vi "Configuration Window.vi"(8 "error in (no error)":errorcluster, 11 "Inst.TC":refnum<class "Inst.TC.lvclass">) -> (0 "error out":errorcluster, 3 "Inst.TC out":refnum<class "Inst.TC.lvclass">)   [LabVIEW 2019, in "Inst.TC.lvclass"]
uses:
  Inst.TC.lvclass
  C:/Program Files (x86)/National Instruments/LabVIEW 2019/vi.lib/JKI/JKI SMO/SMO/SMO.lvclass
  Inst.TC.lvclass/Inst.TC.ctl
  FP-TC-Shared/FP-TC-Shared.lvclass/FP-TC-Shared.ctl
  <userlib>/LevyLab/Debug/Attribute.Debug/DebugBehavior.ctl
  FP-TC-Shared/FP-TC-Shared.lvclass
  <userlib>/LevyLab/Debug/Debug.lvlib
  <userlib>/LevyLab/Debug/Attribute.Debug/Attribute.Debug.lvclass
panel:
  in  "Debug Mode? [F]":bool
  in  "Paths":string
  in  "LC Type":u16(ring) items=["CF_TC", "CF_TC_Z", "MNK_TC", "MNK_TC_Z"]
  in  "Cancel":bool
  in  "OK":bool
  # "Confirm or Make Changes:"
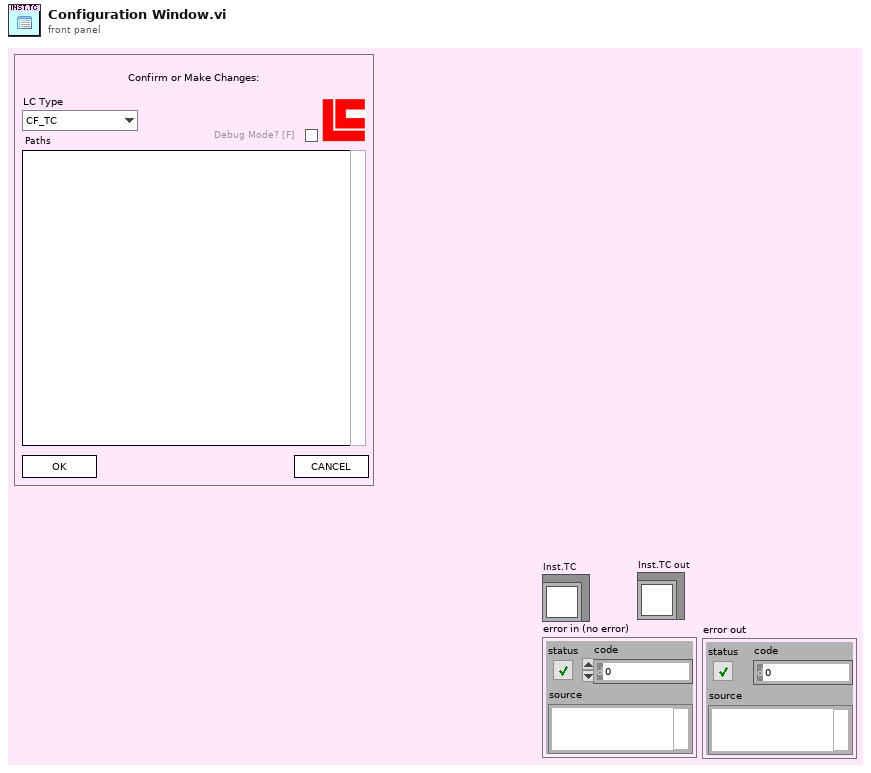
[diagram p1: front panel]
types:
  T1 = enum32{"Invalid", "Standard", "Closed", "Hidden", "Minimized", "Maximized"}
  T2 = enum32{"invalid app kind", "Development System", "Run Time System", "Student Edition", "Embedded LabVIEW", "Evaluation", "Custom"}
  T3 = typedef "Debug.lvlib/Attribute.Debug.lvclass/DebugBehavior.ctl" = enum16{"Normal", "Debug"}
  T4 = cluster{"Core":cluster{"Current VI Reference":refnum<vi>, "Close Panel on Exit?":bool}, "Inst.TC":refnum<class "Inst.TC.lvclass">}
  T5 = typedef "FP-TC-Shared.lvclass/LC Type--Enum.ctl" = enum16{"CF_FP", "CF_TC", "CF_TC_Z", "MNK_FP", "MNK_TC", "MNK_TC_Z", "unknown"}
  T6 = cluster{"Current VI Reference":refnum<vi>, "Close Panel on Exit?":bool}
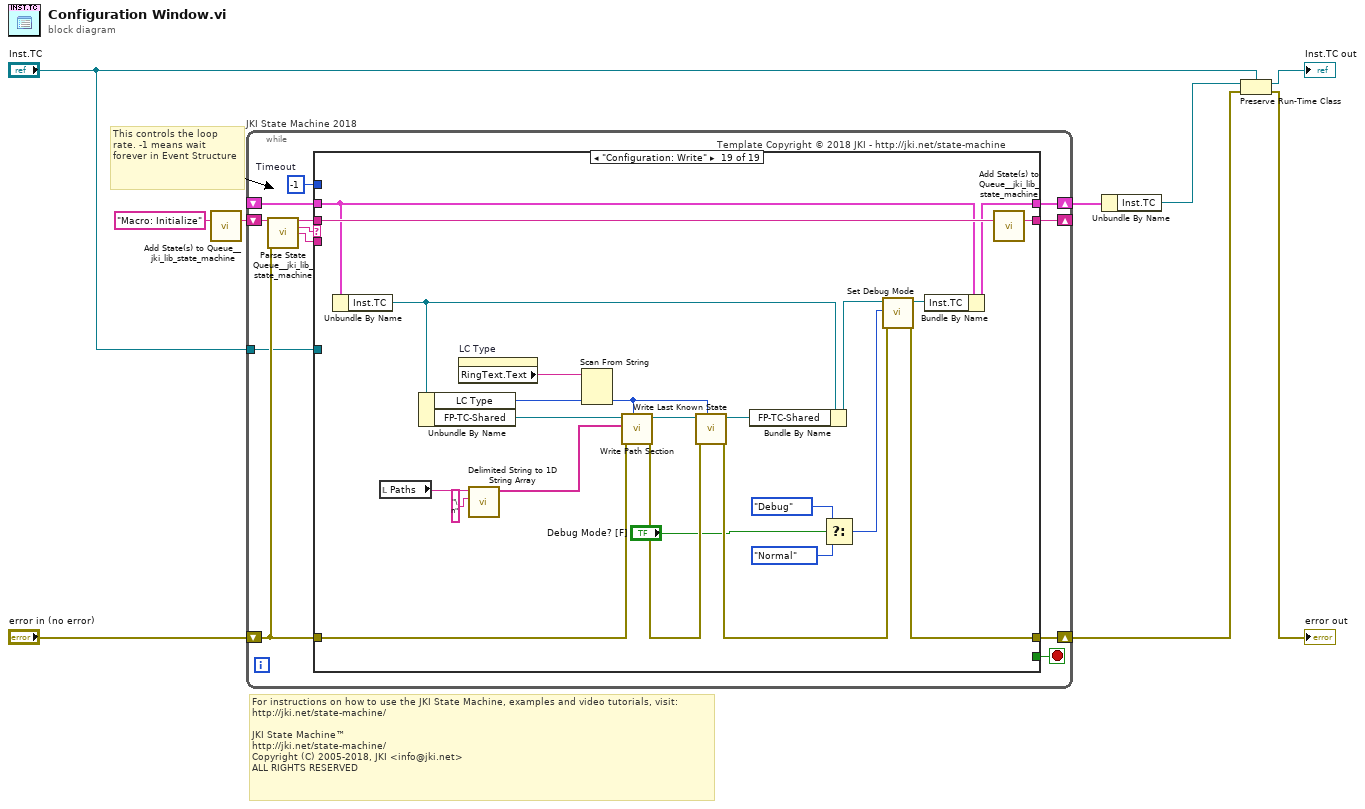
[diagram p0: block diagram]
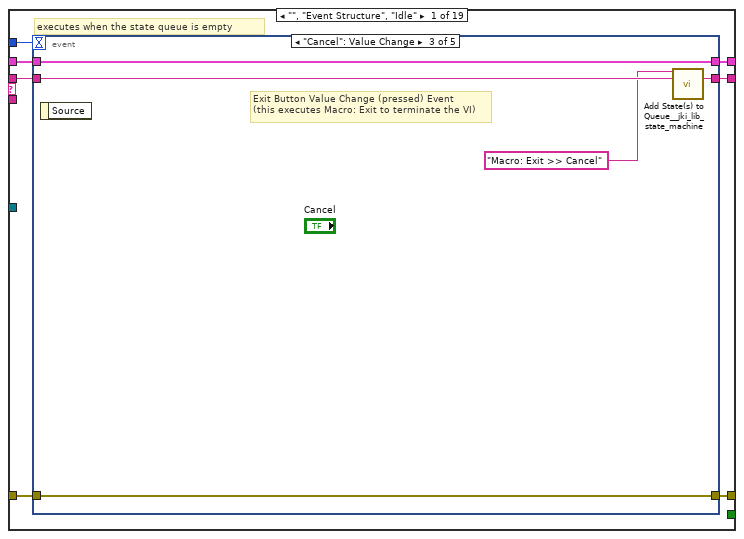
[diagram p2: hidden frame]
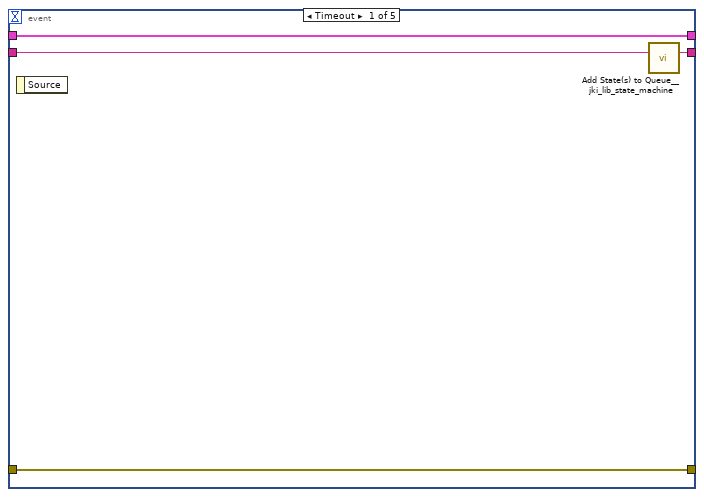
[diagram p3: hidden frame]
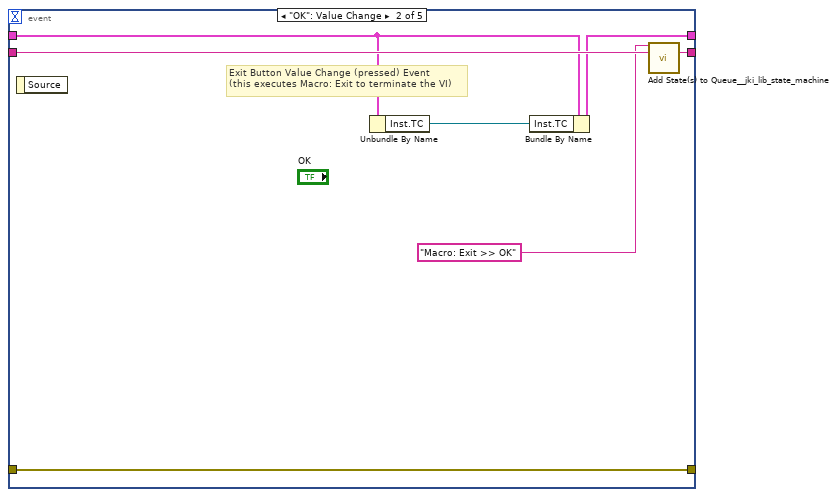
[diagram p4: hidden frame]
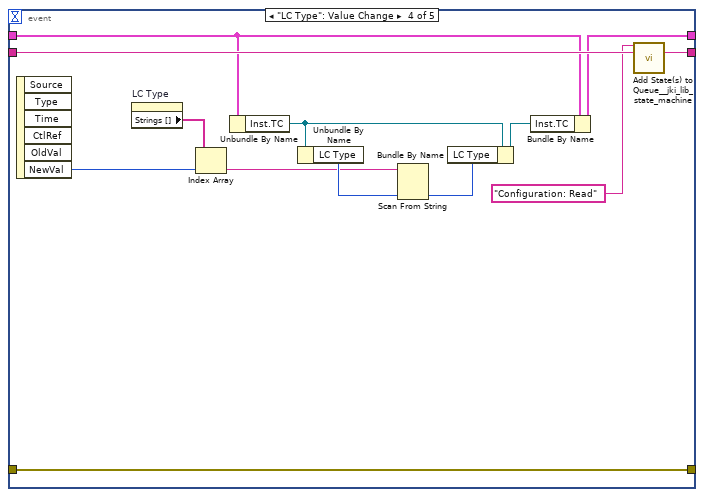
[diagram p5: hidden frame]
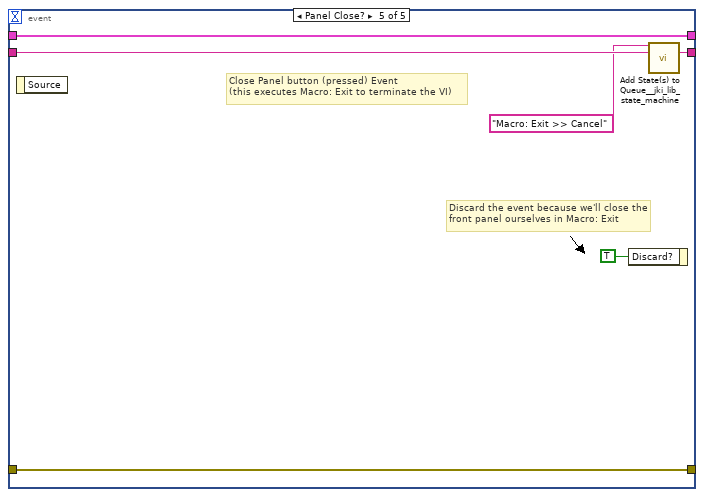
[diagram p6: hidden frame]
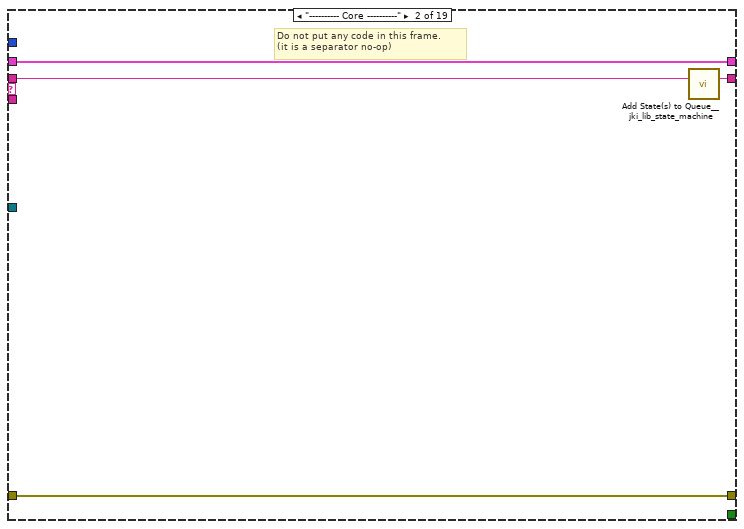
[diagram p7: hidden frame]
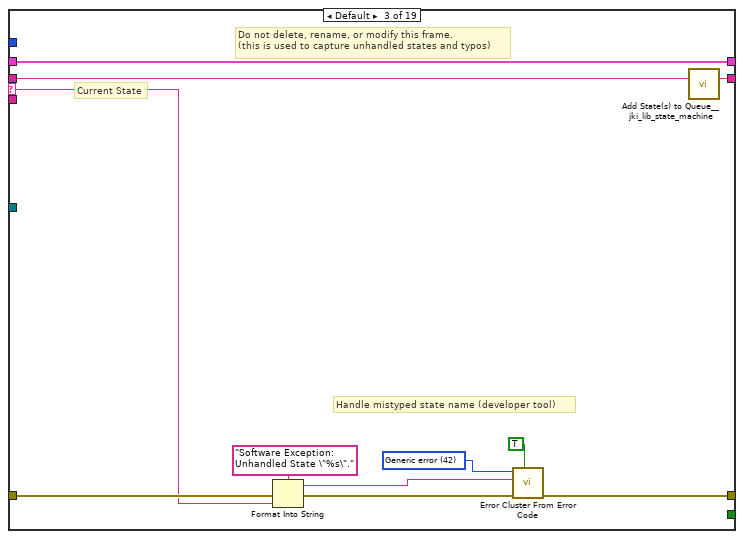
[diagram p8: hidden frame]
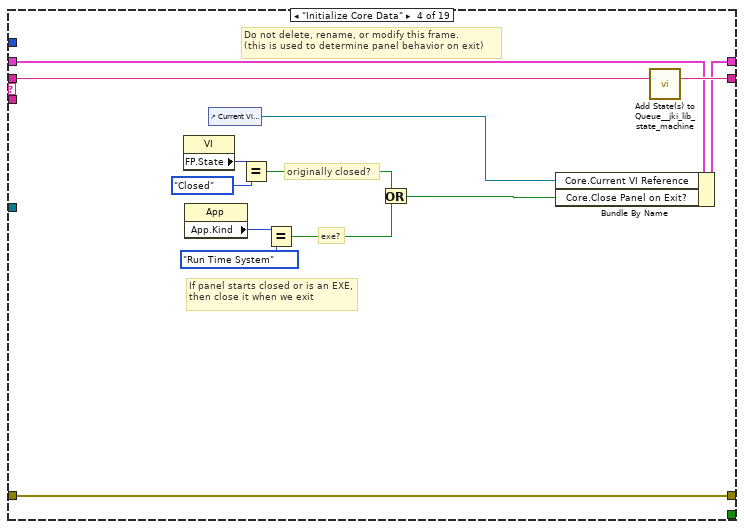
[diagram p9: hidden frame]
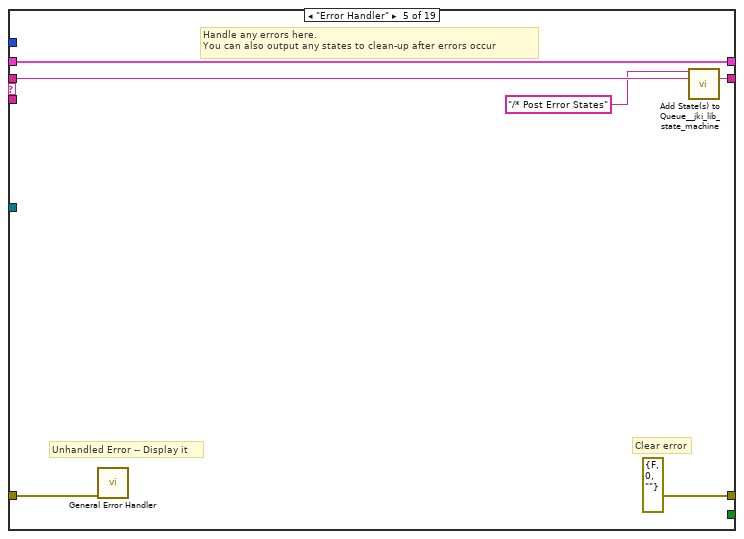
[diagram p10: hidden frame]
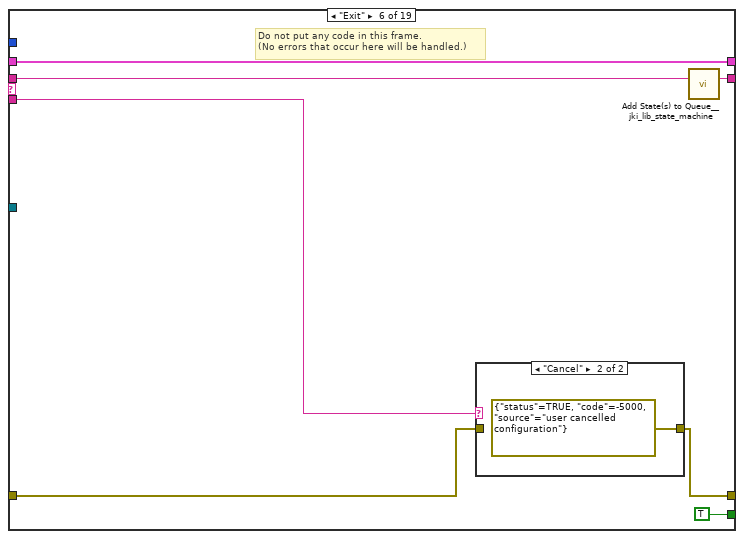
[diagram p11: hidden frame]
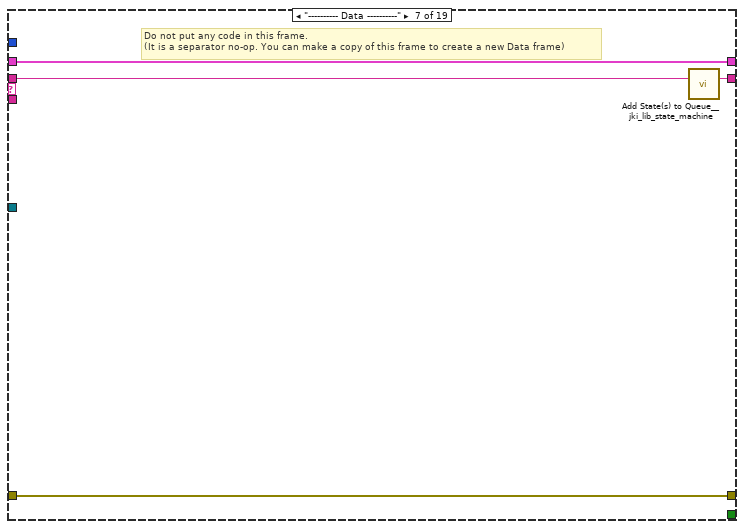
[diagram p13: hidden frame]
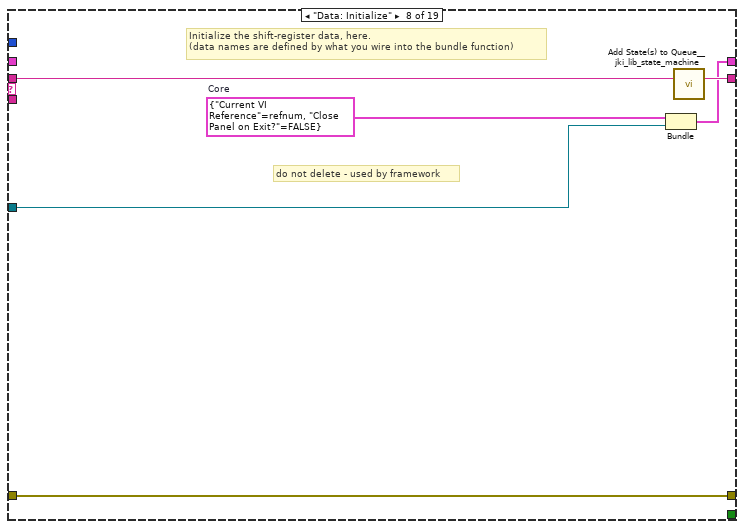
[diagram p14: hidden frame]
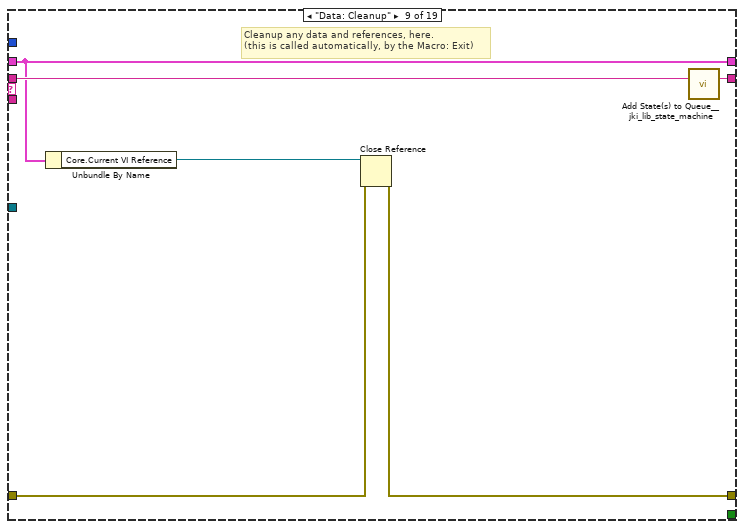
[diagram p15: hidden frame]
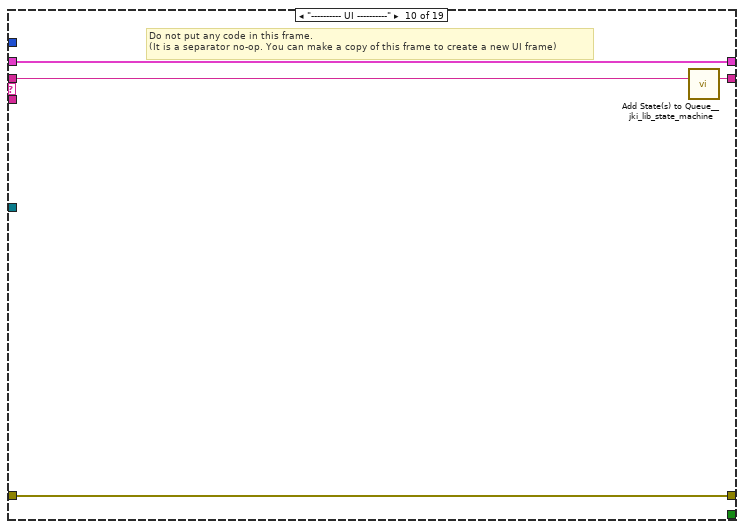
[diagram p16: hidden frame]
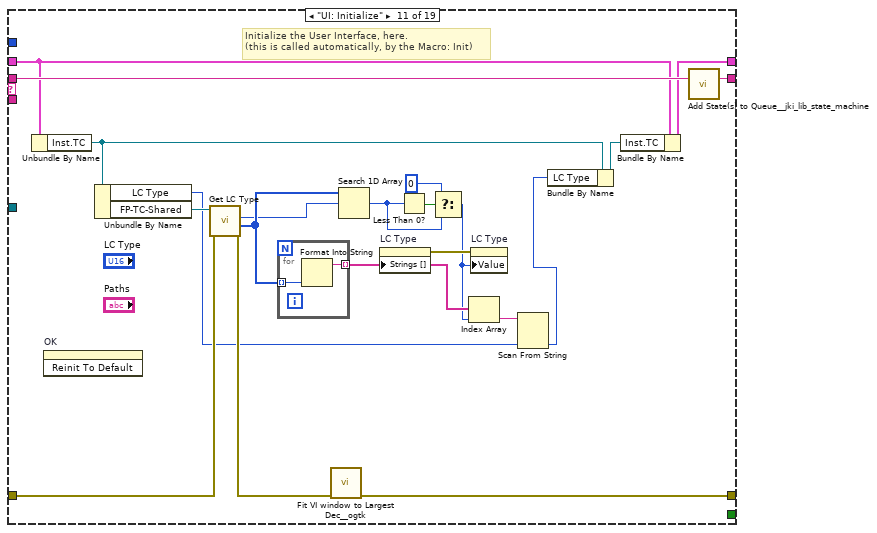
[diagram p17: hidden frame]
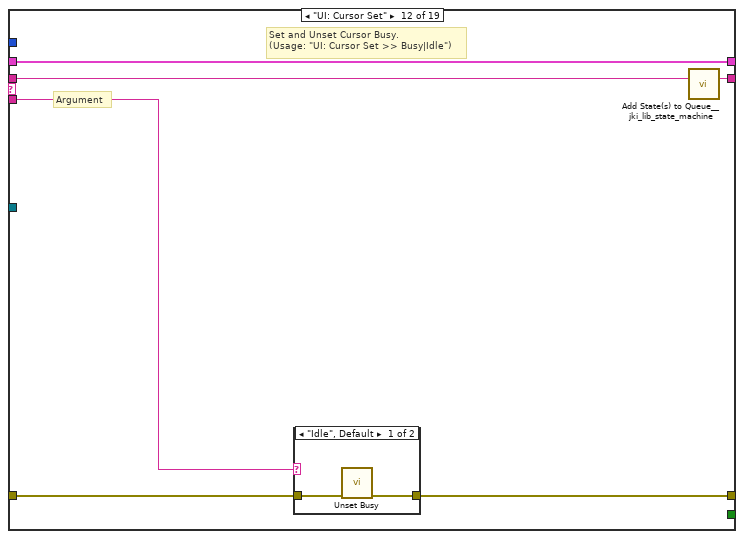
[diagram p18: hidden frame]
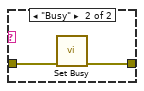
[diagram p19: hidden frame]
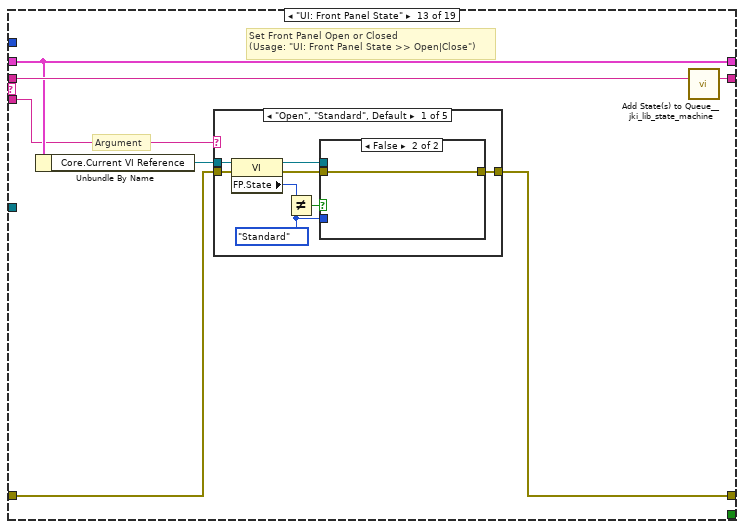
[diagram p20: hidden frame]
diagram:
  # "For instructions on how to use the JKI State Machine, examples and video tutorials, visit:\nhttp://jki.net/state-machine/\n\nJKI State Machine™\nhttp://jki.net/state-machine/\nCopyright (C) 2005-2018, JKI <info@jki.net>\nALL RIGHTS RESERVED"
  # "This controls the loop rate. -1 means wait forever in Event Structure"
  n1 = call <vilib>:"Add State(s) to Queue__jki_lib_state_machine.vi"("State(s) in (\"\")"="Macro: Initialize") -> ("States Out"=w6:string)  [unwired: 14 in]
  n2 = while "JKI State Machine 2018" {
    shift-right: [w14] -> w3
    shift-left: _ -> [w13]
    shift-right: [w17] -> w4
    shift-left: "error in (no error)" -> [w11]
    shift-right: [w16] -> _
    shift-left: w6 -> [w18]
    tunnel: "Inst.TC" -> [w10]
    stop <- w15 stop-if-true
    w12 = -1  # Timeout
    # "Template Copyright © 2018 JKI - http://jki.net/state-machine"
    n3 = call <vilib>:"Parse State Queue__jki_lib_state_machine.vi"("State Queue"=w18, "Error In (no error)"=w11) -> ("Remaining States"=w20:string, "Current State"=w21:string, "Arguments"=w19:string)  [unwired: 11 in]
    n4 = case shown="\"Configuration: Write\"" w21 {
      selector: w21 -> [_ _ w68 _ _ _ _ _ _ _ _ _ _ _ _ _ _ _ _]
      tunnel: w20 -> [w28 w67 w72 w91 w97 w104 w110 w116 w122 w126 w147 w155 w166 w235 w240 w255 w261 w275 w299]
      tunnel: w19 -> [_ _ _ _ _ w100 _ _ _ _ _ w150 w160 _ _ w241 _ _ _]
      tunnel: w13 -> [w26 w64 w70 w84 w94 w102 w107 _ w117 w123 w144 w153 w162 w232 w237 w252 w258 w272 w296]
      tunnel: [w25 w65 w74 w88 errorcluster {"status"=FALSE, "code"=0, "source"=""} ("error out") w98 w108 w112 w118 w124 w145 w151 w163 w233 w238 w253 w259 w267 w278] -> w17
      tunnel: w11 -> [w24 w65 w73 w88 w93 w99 w108 w112 w119 w124 w134 w152 w164 w233 w238 w253 w259 w268 w290]
      tunnel: [w27 w66 w71 w90 w96 w103 w109 w115 w121 w125 w146 w154 w165 w234 w239 w254 w260 w274 w298] -> w16
      tunnel: [_ _ _ _ _ TRUE _ _ _ _ _ _ _ _ _ _ _ _ _] -> w15
      tunnel: [w23 w64 w70 w89 w94 w102 w107 w114 w117 w123 w143 w153 w162 w232 w237 w252 w258 w273 w297] -> w14
      tunnel: w12 -> [w22 _ _ _ _ _ _ _ _ _ _ _ _ _ _ _ _ _ _]
      tunnel: w10 -> [_ _ _ _ _ _ _ w111 _ _ _ _ _ _ _ _ _ _ _]
      frame "", "Event Structure", "Idle" {
        # "executes when the state queue is empty"
        n5 = event shown="[2] \"Cancel\": Value Change" {
          selector: _ -> [_ _ _ _ _]
          dyn-events: _ -> [_ _ _ _ _]
          timeout: w22 -> [_ _ _ _ _]
          tunnel: w28 -> [w32 w39 w44 w56 w63]
          tunnel: [w31 w38 w43 w57 w62] -> w27
          tunnel: w26 -> [w29 w35 w40 w53 w60]
          tunnel: [w30 w37 w42 w51 w61] -> w25
          tunnel: w24 -> [w30 w37 w42 w51 w61]
          tunnel: [w29 w36 w40 w54 w60] -> w23
          event Timeout {
            n6 = event-data() -> ()  [unwired: 1 in, 1 out]
            n7 = call <vilib>:"Add State(s) to Queue__jki_lib_state_machine.vi"("State(s) in (\"\")"=w32) -> ("States Out"=w31:string)  [unwired: 14 in]
          }
          event "OK": Value Change {
            # "Exit Button Value Change (pressed) Event\n(this executes Macro: Exit to terminate the VI)"
            n8 = event-data() -> ()  [unwired: 1 in, 1 out]
            n9 = Unbundle By Name(w35) -> ("Inst.TC"=w33:refnum<class "Inst.TC.lvclass">)
            n10 = Bundle By Name(cluster=w35, "Inst.TC"=w33) -> (w36:T4)
            n11 = call <vilib>:"Add State(s) to Queue__jki_lib_state_machine.vi"("State(s) in Front (\"\")"="Macro: Exit >> OK", "State(s) in (\"\")"=w39) -> ("States Out"=w38:string)  [unwired: 13 in]
          }
          event "Cancel": Value Change {
            # "Exit Button Value Change (pressed) Event\n(this executes Macro: Exit to terminate the VI)"
            n12 = event-data() -> ()  [unwired: 1 in, 1 out]
            n13 = call <vilib>:"Add State(s) to Queue__jki_lib_state_machine.vi"("State(s) in Front (\"\")"="Macro: Exit >> Cancel", "State(s) in (\"\")"=w44) -> ("States Out"=w43:string)  [unwired: 13 in]
          }
          event "LC Type": Value Change {
            n14 = event-data() -> ("NewVal"=w49:u16)  [unwired: 1 in, 5 out]
            n15 = property on="LC Type" class="Ring (strict)"() -> ("Strings []"=w50:string[])  [unwired: 2 in, 2 out]
            n16 = Index Array(array=w50, index=w49) -> (element=w45:string)
            n17 = Unbundle By Name(w53) -> ("Inst.TC"=w48:refnum<class "Inst.TC.lvclass">)
            n18 = Unbundle By Name(w48) -> ("LC Type"=w47:T5)
            n19 = Scan From String(input string=w45, default 1=w47) -> (output 1=w46:T5)  [unwired: 3 in, 3 out]
            n20 = Bundle By Name(cluster=w48, "LC Type"=w46) -> (w52:refnum<class "Inst.TC.lvclass">)
            n21 = Bundle By Name(cluster=w53, "Inst.TC"=w52) -> (w54:T4)
            n22 = call <vilib>:"Add State(s) to Queue__jki_lib_state_machine.vi"("State(s) in Front (\"\")"="Configuration: Read" ("State(s) in Front (\"\")"), "State(s) in (\"\")"=w56) -> ("States Out"=w57:string)  [unwired: 13 in]
          }
          event Panel Close? {
            # "Discard the event because we'll close the front panel ourselves in Macro: Exit"
            # "Close Panel button (pressed) Event\n(this executes Macro: Exit to terminate the VI)"
            n23 = event-data() -> ()  [unwired: 1 in, 1 out]
            n24 = event-data("Discard?"=TRUE) -> ()  [unwired: 1 in, 1 out]
            n25 = call <vilib>:"Add State(s) to Queue__jki_lib_state_machine.vi"("State(s) in Front (\"\")"="Macro: Exit >> Cancel", "State(s) in (\"\")"=w63) -> ("States Out"=w62:string)  [unwired: 13 in]
          }
        }
      }
      frame "---------- Core ----------" {
        # "Do not put any code in this frame.\n(it is a separator no-op)"
        n26 = call <vilib>:"Add State(s) to Queue__jki_lib_state_machine.vi"("State(s) in (\"\")"=w67) -> ("States Out"=w66:string)  [unwired: 14 in]
      }
      frame Default {
        w77 = 42 items=["No error", "Argument error", "Memory is full", "Out of zone", "End of file", "File already open", "Generic file I/O error", "File not found", "File permission error", "Disk is full", "Duplicate path", "Too many files open", "System feature not enabled", "Resource file not found", "Cannot add resource", "Resource not found", "Image not found", "Image memory error", "Pen does not exist", "Config type invalid", "Config token not found", "Config parse error", "Config memory error", "Bad external code format", "Bad external code offset", "External code not present", "Null window", "Destroy window error", "Null menu", "Print aborted", "Bad print record", "Print driver error", "Windows error during printing", "Memory error during printing", "Print dialog error", "Generic print error", "Invalid device refnum", "Device not found", "Device parameter error", "Device unit error", "Cannot open device", "Device call aborted", "Generic error", "Cancelled by user", "Object ID too low", "Object ID too high", "Object not in heap", "Unknown heap", "Unknown object (invalid DefProc)", "Unknown object (DefProc not in table)", "Message out of range", "Invalid (null) method", "Unknown message", "Manager call not supported", "Bad address", "Network operation in progress", "Network operation timed out", "Connection is busy", "Network attribute not supported", "Network error", "Address in use", "System out of memory", "Connection aborted", "Connection refused", "Not connected", "Already connected", "Connection closed", "Initialization error (interapplication manager)", "Bad occurrence", "Wait on unbound occurrence handler", "Occurrence queue overflow", "Datalog type conflict", "Unused", "Unrecognized type (interapplication manager)", "Memory corrupt", "Failed to make temporary DLL", "Old CIN version", "Drag socket not found", "Failed to load drop-object", "Failed to register OLE object", "Failed to release OLE object", "Format specifier type mismatch", "Unknown format specifier", "Too few format specifiers", "Too many format specifiers", "Scan failed", "Newer CIN version", "Error converting to variant", "Runtime menu error", "Password tampered", "Variant attribute not found", "Incompatible variant data type", "Event data is not available", "Event Store is not present", "Occurrence is not found", "Event Queue is not created", "Event info is not available", "Refnum passed is NULL", "Error retrieving Class GUID", "Error retrieving CoClass GUID", "Error retrieving TypeLib GUID.", "Bad built application magic bytes.", "Specific driver is different from the specific driver associated with the Logical Name.", "There is no session opened to the class driver.", "Max Error", "MAX - Error with config objects", "MAX - Error loading configuration", "MAX - Group not supported"]
        # "Current State"
        # "Do not delete, rename, or modify this frame.\n(this is used to capture unhandled states and typos)"
        # "Handle mistyped state name (developer tool)"
        n27 = Format Into String(format string="Software Exception: Unhandled State \"%s\"." ("message"), error in=w73, w68) -> (resulting string=w76:string, error out=w75:errorcluster)  [unwired: 1 in]
        n28 = call <vilib>:"Error Cluster From Error Code.vi"("show call chain? (False)"=TRUE, "error in (no error)"=w75, "error message (\"\")"=w76, "error code (0)"=w77) -> ("error out"=w74:errorcluster)  [unwired: 5 in]
        n29 = call <vilib>:"Add State(s) to Queue__jki_lib_state_machine.vi"("State(s) in (\"\")"=w72) -> ("States Out"=w71:string)  [unwired: 14 in]
      }
      frame "Initialize Core Data" {
        # "Do not delete, rename, or modify this frame.\n(this is used to determine panel behavior on exit)"
        # "originally closed?"
        # "exe?"
        # "If panel starts closed or is an EXE, then close it when we exit"
        n30 = property class="VI"() -> ("FP.State"=w81:T1)  [unwired: 2 in, 2 out]
        n31 = property class="App"() -> ("App.Kind"=w87:T2)  [unwired: 2 in, 2 out]
        n32 = control-ref of="Current VI Reference"() -> (w82:refnum<vi>)
        n33 = Equal?(x=w81, y=T1."Closed" ("Front Panel Window:State")) -> (x = y?=w79:bool)
        n34 = Equal?(x=w87, y=T2."Run Time System" ("Application:Kind")) -> (x = y?=w85:bool)
        n35 = Or(x=w79, y=w85) -> (x .or. y?=w83:bool)
        n36 = Bundle By Name(cluster=w84, "Core.Current VI Reference"=w82, "Core.Close Panel on Exit?"=w83) -> (w89:T4)
        n37 = call <vilib>:"Add State(s) to Queue__jki_lib_state_machine.vi"("State(s) in (\"\")"=w91) -> ("States Out"=w90:string)  [unwired: 14 in]
      }
      frame "Error Handler" {
        # "Unhandled Error -- Display it"
        # "Handle any errors here.\nYou can also output any states to clean-up after errors occur"
        # "Clear error"
        n38 = call <vilib>:"General Error Handler.vi"("error in (no error)"=w93) -> ()  [unwired: 10 in, 5 out]
        n39 = call <vilib>:"Add State(s) to Queue__jki_lib_state_machine.vi"("State(s) in Front (\"\")"="/* Post Error States", "State(s) in (\"\")"=w97) -> ("States Out"=w96:string)  [unwired: 13 in]
      }
      frame "Exit" {
        # "Do not put any code in this frame.\n(No errors that occur here will be handled.)"
        n40 = case shown="\"Cancel\"" w100 {
          tunnel: w99 -> [w105 _]
          tunnel: [w105 errorcluster {"status"=TRUE, "code"=-5000, "source"="user cancelled configuration"} ("error in (no error)")] -> w98
          frame "OK", Default {
          }
          frame "Cancel" {
          }
        }
        n41 = call <vilib>:"Add State(s) to Queue__jki_lib_state_machine.vi"("State(s) in (\"\")"=w104) -> ("States Out"=w103:string)  [unwired: 14 in]
      }
      frame "---------- Data ----------" {
        # "Do not put any code in this frame.\n(It is a separator no-op. You can make a copy of this frame to create a new Data frame)"
        n42 = call <vilib>:"Add State(s) to Queue__jki_lib_state_machine.vi"("State(s) in (\"\")"=w110) -> ("States Out"=w109:string)  [unwired: 14 in]
      }
      frame "Data: Initialize" {
        w113 = T6 {"Current VI Reference"=refnum, "Close Panel on Exit?"=FALSE}  # Core
        # "do not delete - used by framework"
        # "Initialize the shift-register data, here.\n(data names are defined by what you wire into the bundle function)"
        n43 = Bundle("Core"=w113, "Inst.TC"=w111) -> (w114:T4)  [unwired: 1 in]
        n44 = call <vilib>:"Add State(s) to Queue__jki_lib_state_machine.vi"("State(s) in (\"\")"=w116) -> ("States Out"=w115:string)  [unwired: 14 in]
      }
      frame "Data: Cleanup" {
        # "Cleanup any data and references, here.\n(this is called automatically, by the Macro: Exit)"
        n45 = Unbundle By Name(w117) -> ("Core.Current VI Reference"=w120:refnum<vi>)
        n46 = Close Reference(reference=w120, error in (no error)=w119) -> (error out=w118:errorcluster)
        n47 = call <vilib>:"Add State(s) to Queue__jki_lib_state_machine.vi"("State(s) in (\"\")"=w122) -> ("States Out"=w121:string)  [unwired: 14 in]
      }
      frame "---------- UI ----------" {
        # "Do not put any code in this frame.\n(It is a separator no-op. You can make a copy of this frame to create a new UI frame)"
        n48 = call <vilib>:"Add State(s) to Queue__jki_lib_state_machine.vi"("State(s) in (\"\")"=w126) -> ("States Out"=w125:string)  [unwired: 14 in]
      }
      frame "UI: Initialize" {
        # "Initialize the User Interface, here.\n(this is called automatically, by the Macro: Init)"
        n49 = Unbundle By Name(w144) -> ("Inst.TC"=w133:refnum<class "Inst.TC.lvclass">)
        n50 = invoke on="OK" class="Bool" method="Reinit To Default"() -> ()  [unwired: 3 in, 3 out]
        n51 = Unbundle By Name(w133) -> ("LC Type"=w128:T5, "FP-TC-Shared"=w136:refnum<class "FP-TC-Shared.lvclass">)
        n52 = call "Get LC Type.vi"("error in (no error)"=w134, "FP-TC-Shared in"=w136) -> ("error out"=w135:errorcluster, "LC Types"=w142:T5[], "LC Type"=w140:T5)  [unwired: 5 in, 2 out]
        n53 = for {
          tunnel: w142 -> [w149] mode=indexing
          tunnel: [w148] -> w131 mode=indexing
          n54 = Format Into String(w149) -> (resulting string=w148:string)  [unwired: 3 in, 1 out]
        }
        n55 = call <userlib>:"Fit VI window to Largest Dec__ogtk.vi"("error in (no error)"=w135) -> ("error out"=w145:errorcluster)  [unwired: 5 in, 1 out]
        n56 = Search 1D Array(1D array=w142, element=w140) -> (index of element=w138:i32)  [unwired: 1 in]
        n57 = property on="LC Type" class="Ring (strict)"("Strings []"=w131) -> (error out=w141:errorcluster)  [unwired: 2 in, 1 out]
        n58 = Less Than 0?(x=w138) -> (x < 0?=w139:bool)
        n59 = Select(t=0, s=w139, f=w138) -> (s? t:f=w130:i32)
        n60 = Index Array(array=w131, index=w130) -> (element=w129:string)
        n61 = property on="LC Type" class="Ring (strict)"(error in=w141, "Value"=w130) -> ()  [unwired: 1 in, 2 out]
        n62 = Scan From String(input string=w129, default 1=w128) -> (output 1=w127:T5)  [unwired: 3 in, 3 out]
        n63 = Bundle By Name(cluster=w133, "LC Type"=w127) -> (w132:refnum<class "Inst.TC.lvclass">)
        n64 = Bundle By Name(cluster=w144, "Inst.TC"=w132) -> (w143:T4)
        n65 = call <vilib>:"Add State(s) to Queue__jki_lib_state_machine.vi"("State(s) in (\"\")"=w147) -> ("States Out"=w146:string)  [unwired: 14 in]
      }
      frame "UI: Cursor Set" {
        # "Argument"
        # "Set and Unset Cursor Busy.\n(Usage: \"UI: Cursor Set >> Busy|Idle\")"
        n66 = case shown="\"Idle\", Default" w150 {
          tunnel: w152 -> [w157 w159]
          tunnel: [w156 w158] -> w151
          frame "Idle", Default {
            n67 = call <vilib>:"Unset Busy.vi"("error in (no error)"=w157) -> ("error out"=w156:errorcluster)  [unwired: 10 in]
          }
          frame "Busy" {
            n68 = call <vilib>:"Set Busy.vi"("error in (no error)"=w159) -> ("error out"=w158:errorcluster)  [unwired: 9 in, 1 out]
          }
        }
        n69 = call <vilib>:"Add State(s) to Queue__jki_lib_state_machine.vi"("State(s) in (\"\")"=w155) -> ("States Out"=w154:string)  [unwired: 14 in]
      }
      frame "UI: Front Panel State" {
        # "Argument"
        # "Set Front Panel Open or Closed\n(Usage: \"UI: Front Panel State >> Open|Close\")"
        n70 = Unbundle By Name(w162) -> ("Core.Current VI Reference"=w161:refnum<vi>)
        n71 = case shown="\"Open\", \"Standard\", Default" w160 {
          tunnel: w164 -> [w172 w187 w198 w211 w224]
          tunnel: [w174 w188 w200 w213 w226] -> w163
          tunnel: w161 -> [w173 w185 w199 w212 w225]
          frame "Open", "Standard", Default {
            w167 = T1."Standard" ("State")
            n72 = property class="VI"(reference=w173, error in=w172) -> (reference out=w170:refnum<vi>, error out=w171:errorcluster, "FP.State"=w169:T1)
            n73 = Not Equal?(x=w169, y=w167) -> (x != y?=w168:bool)
            n74 = case shown="False" w168 {
              tunnel: [w178 w180] -> w174
              tunnel: w171 -> [w177 w180]
              tunnel: w170 -> [w176 _]
              tunnel: w167 -> [w175 _]
              frame True {
                n75 = invoke class="VI" method="FP.Open"(reference=w176, error in=w177, "Activate"=TRUE, "State"=w175) -> (error out=w178:errorcluster)  [unwired: 1 in, 4 out]
              }
              frame False {
              }
            }
          }
          frame "Close", "Closed" {
            n76 = property class="VI"(reference=w185, error in=w187) -> (reference out=w184:refnum<vi>, error out=w186:errorcluster, "FP.State"=w182:T1)
            n77 = Not Equal?(x=w182, y=T1."Closed" ("Front Panel Window:State")) -> (x != y?=w181:bool)
            n78 = case shown="True" w181 {
              tunnel: [w189 w192] -> w188
              tunnel: w186 -> [w189 w191]
              tunnel: w184 -> [_ w190]
              frame False {
              }
              frame True {
                n79 = invoke class="VI" method="FP.Close"(reference=w190, error in=w191) -> (error out=w192:errorcluster)  [unwired: 1 in, 2 out]
              }
            }
          }
          frame "Hidden", "Hide" {
            w193 = T1."Hidden" ("State")
            n80 = property class="VI"(reference=w199, error in=w198) -> (reference out=w196:refnum<vi>, error out=w197:errorcluster, "FP.State"=w195:T1)
            n81 = Not Equal?(x=w195, y=w193) -> (x != y?=w194:bool)
            n82 = case shown="True" w194 {
              tunnel: [w204 w205] -> w200
              tunnel: w197 -> [w203 w205]
              tunnel: w196 -> [w202 _]
              tunnel: w193 -> [w201 _]
              frame True {
                n83 = invoke class="VI" method="FP.Open"(reference=w202, error in=w203, "State"=w201) -> (error out=w204:errorcluster)  [unwired: 2 in, 4 out]
              }
              frame False {
              }
            }
          }
          frame "Minimize", "Minimized" {
            w206 = T1."Minimized" ("State")
            n84 = property class="VI"(reference=w212, error in=w211) -> (reference out=w209:refnum<vi>, error out=w210:errorcluster, "FP.State"=w208:T1)
            n85 = Not Equal?(x=w208, y=w206) -> (x != y?=w207:bool)
            n86 = case shown="True" w207 {
              tunnel: [w217 w218] -> w213
              tunnel: w210 -> [w216 w218]
              tunnel: w209 -> [w215 _]
              tunnel: w206 -> [w214 _]
              frame True {
                n87 = invoke class="VI" method="FP.Open"(reference=w215, error in=w216, "State"=w214) -> (error out=w217:errorcluster)  [unwired: 2 in, 4 out]
              }
              frame False {
              }
            }
          }
          frame "Maximize", "Maximized" {
            w219 = T1."Maximized" ("State")
            n88 = property class="VI"(reference=w225, error in=w224) -> (reference out=w222:refnum<vi>, error out=w223:errorcluster, "FP.State"=w221:T1)
            n89 = Not Equal?(x=w221, y=w219) -> (x != y?=w220:bool)
            n90 = case shown="True" w220 {
              tunnel: [w230 w231] -> w226
              tunnel: w223 -> [w229 w231]
              tunnel: w222 -> [w228 _]
              tunnel: w219 -> [w227 _]
              frame True {
                n91 = invoke class="VI" method="FP.Open"(reference=w228, error in=w229, "State"=w227) -> (error out=w230:errorcluster)  [unwired: 2 in, 4 out]
              }
              frame False {
              }
            }
          }
        }
        n92 = call <vilib>:"Add State(s) to Queue__jki_lib_state_machine.vi"("State(s) in (\"\")"=w166) -> ("States Out"=w165:string)  [unwired: 14 in]
      }
      frame "---------- Macro ----------" {
        # "Do not put any code in this frame.\n(It is a separator no-op. You can make a copy of this frame to create a new Macro frame)"
        n93 = call <vilib>:"Add State(s) to Queue__jki_lib_state_machine.vi"("State(s) in (\"\")"=w235) -> ("States Out"=w234:string)  [unwired: 14 in]
      }
      frame "Macro: Initialize" {
        w236 = "Data: Initialize\nInitialize Core Data\nUI: Initialize\nUI: Front Panel State >> Open\nConfiguration: Read"  # Data: Initialize Initialize Core Data UI: Initialize UI: Front Panel State >> Open Configuration: Read
        # "Initialization Macro\n(This is called once, when the VI starts)"
        n94 = call <vilib>:"Add State(s) to Queue__jki_lib_state_machine.vi"("State(s) in Front (\"\")"=w236, "State(s) in (\"\")"=w240) -> ("States Out"=w239:string)  [unwired: 13 in]
      }
      frame "Macro: Exit" {
        # "Exit Macro\n(This is called once, when the VI exits)"
        n95 = Unbundle By Name(w252) -> ("Core.Close Panel on Exit?"=w251:bool)
        n96 = case shown="Default" w241 {
          tunnel: ["" "Configuration: Write"] -> w246
          frame Default {
          }
          frame "OK" {
          }
        }
        n97 = call <vilib>:"Build State String with Arguments__JKI_lib_State_Machine.vi"("Arguments (\"\")"=w241, "State"="Exit") -> ("State with Arguments"=w243:string)  [unwired: 4 in]
        n98 = Select(t="UI: Front Panel State >> Close", s=w251, f="") -> (s? t:f=w248:string)
        n99 = call <vilib>:"Add State(s) to Queue__jki_lib_state_machine.vi"("State(s) in Front (\"\")"="Data: Cleanup", "State(s) at Back (\"\")"=w243) -> ("States Out"=w242:string)  [unwired: 13 in]
        n100 = call <vilib>:"Add State(s) to Queue__jki_lib_state_machine.vi"("State(s) in Front (\"\")"=w246, "State(s) in (\"\")"=w248, "State(s) at Back (\"\")"=w242) -> ("States Out"=w247:string)  [unwired: 12 in]
        n101 = call <vilib>:"Add State(s) to Queue__jki_lib_state_machine.vi"("State(s) in Front (\"\")"=w247, "State(s) in (\"\")"=w255) -> ("States Out"=w254:string)  [unwired: 13 in]
      }
      frame "---------- Configuration ----------" {
        # "Template Separator\n(You can make a copy of, or modify, this frame)"
        n102 = call <vilib>:"Add State(s) to Queue__jki_lib_state_machine.vi"("State(s) in (\"\")"=w261) -> ("States Out"=w260:string)  [unwired: 14 in]
      }
      frame "Configuration: Read" {
        # "Your code here.\n(You can make a copy of, or modify, this frame)"
        n103 = Unbundle By Name(w272) -> ("Inst.TC"=w265:refnum<class "Inst.TC.lvclass">)
        n104 = Unbundle By Name(w265) -> ("LC Type"=w271:T5, "FP-TC-Shared"=w266:refnum<class "FP-TC-Shared.lvclass">)
        n105 = call "Read Path Section.vi"("LC Type"=w271, "error in (no error)"=w268, "FP-TC-Shared in"=w266) -> ("error out"=w267:errorcluster, "Paths"=w262:string[], "FP-TC-Shared out"=w264:refnum<class "FP-TC-Shared.lvclass">)  [unwired: 6 in]
        n106 = Bundle By Name(cluster=w265, "FP-TC-Shared"=w264) -> (w263:refnum<class "Inst.TC.lvclass">)
        n107 = call <vilib>:"1D String Array to Delimited String.vi"("delimiter"="\n", "string array"=w262) -> ("delimited string"=w270:string)  [unwired: 9 in]
        n108 = local write "Paths"(w270) -> ()
        n109 = Bundle By Name(cluster=w272, "Inst.TC"=w263) -> (w273:T4)
        n110 = call <vilib>:"Add State(s) to Queue__jki_lib_state_machine.vi"("State(s) in (\"\")"=w275) -> ("States Out"=w274:string)  [unwired: 14 in]
      }
      frame "Configuration: Write" {
        n111 = Unbundle By Name(w296) -> ("Inst.TC"=w288:refnum<class "Inst.TC.lvclass">)
        n112 = local read "Paths"() -> (w286:string)
        n113 = Unbundle By Name(w288) -> ("LC Type"=w294:T5, "FP-TC-Shared"=w293:refnum<class "FP-TC-Shared.lvclass">)
        n114 = property on="LC Type" class="Ring (strict)"() -> ("RingText.Text"=w295:string)  [unwired: 2 in, 2 out]
        n115 = call <vilib>:"Delimited String to 1D String Array.vi"("delimiter"="\n", "delimited string"=w286) -> ("string array"=w284:string[])  [unwired: 9 in]
        n116 = Scan From String(input string=w295, default 1=w294) -> (output 1=w291:T5)  [unwired: 3 in, 3 out]
        n117 = call "Write Path Section.vi"("LC Type"=w291, "error in (no error)"=w290, "paths"=w284, "FP-TC-Shared in"=w293) -> ("error out"=w289:errorcluster, "FP-TC-Shared out"=w292:refnum<class "FP-TC-Shared.lvclass">)  [unwired: 6 in]
        n118 = call "Write Last Known State.vi"("LC Type"=w291, "error in (no error)"=w289, "FP-TC-Shared in"=w292) -> ("error out"=w279:errorcluster, "FP-TC-Shared out"=w287:refnum<class "FP-TC-Shared.lvclass">)  [unwired: 7 in]
        n119 = Bundle By Name(cluster=w288, "FP-TC-Shared"=w287) -> (w281:refnum<class "Inst.TC.lvclass">)
        n120 = Select(t=DebugBehavior."Debug" ("Behavior"), s="Debug Mode? [F]", f=DebugBehavior."Normal" ("Behavior")) -> (s? t:f=w276:T3)
        n121 = call <userlib>:"Set Debug Mode.vi"("error in (no error)"=w279, "Behavior"=w276, "SMO"=w281) -> ("error out"=w278:errorcluster, "SMO out"=w280:refnum<class "Inst.TC.lvclass">)  [unwired: 7 in]
        n122 = Bundle By Name(cluster=w296, "Inst.TC"=w280) -> (w297:T4)
        n123 = call <vilib>:"Add State(s) to Queue__jki_lib_state_machine.vi"("State(s) in (\"\")"=w299) -> ("States Out"=w298:string)  [unwired: 14 in]
      }
    }
  }
  n124 = Unbundle By Name(w3) -> ("Inst.TC"=w2:refnum<class "Inst.TC.lvclass">)
  n125 = Preserve Run-Time Class(object in=w2, error in=w4, 2:"Inst.TC") -> (object out=→"Inst.TC out":refnum<class "Inst.TC.lvclass">, error out=→"error out":errorcluster)
